vi "EX7-1_DC motor control.vi"() -> ()   [LabVIEW 2011]
uses:
  <vilib>/LabVIEW Interface for Arduino/LabVIEW Interface for Arduino.lvlib
panel:
  out "Ready?":bool
  in  "stop":bool
  in  "Selection":T1(radio)
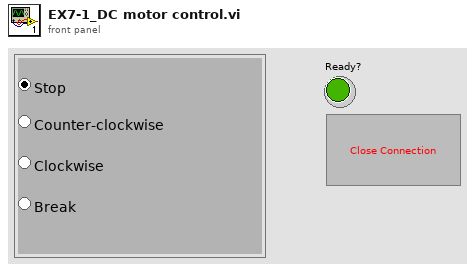
[diagram p1: front panel]
types:
  T1 = enum32{"Stop", "Clockwise", "Counter-clockwise", "Break"}
  T2 = typedef "LabVIEW Interface for Arduino.lvlib/Arduino Resource.ctl" = cluster{"VISA resource":refnum<visa-resource-name>, "Board Type":T3, "Connection Type":enum8{"USB / Serial"}, "Bytes Per Packet (15)":u8}
  T3 = typedef "LabVIEW Interface for Arduino.lvlib/Board Type.ctl" = enum16{"Uno", "Dimuelanove w/Atmega 328", "Mega 2560"}
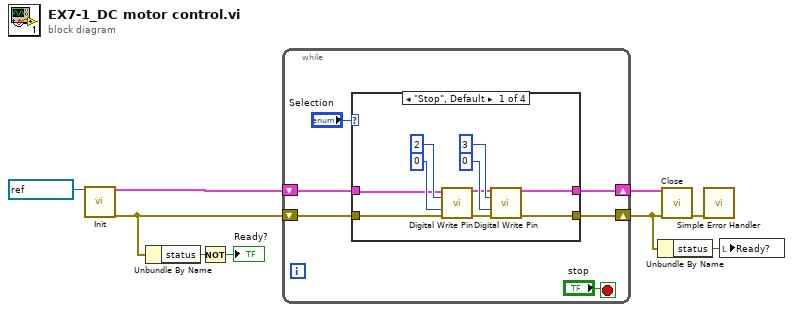
[diagram p0: block diagram]
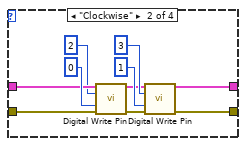
[diagram p2: hidden frame]
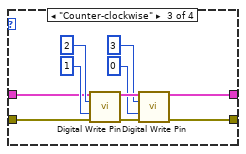
[diagram p3: hidden frame]
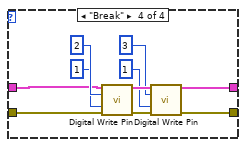
[diagram p4: hidden frame]
diagram:
  n1 = call <vilib>:"Init.vi"("VISA resource"=refnum<visa-resource-name> "COM9") -> ("Arduino Resource"=w8:T2, "error out"=w3:errorcluster)  [unwired: 17 in]
  n2 = Unbundle By Name(w3) -> ("status"=w4:bool)
  n3 = Not(x=w4) -> (.not. x?=→"Ready?":bool)
  n4 = while {
    shift-right: [w12] -> w7
    shift-left: w8 -> [w14]
    shift-right: [w11] -> w2
    shift-left: w3 -> [w13]
    stop <- "stop" stop-if-true
    n5 = case shown="\"Stop\", Default" "Selection" {
      tunnel: w14 -> [w20 w30 w39 w49]
      tunnel: w13 -> [w19 w29 w38 w48]
      tunnel: [w18 w28 w37 w47] -> w12
      tunnel: [w17 w27 w36 w46] -> w11
      frame "Stop", Default {
        n6 = call <vilib>:"Digital Write Pin.vi"("Arduino Resource"=w20, "Digital I/O Pin (0)"=u8 2, "Value (0)"=u8 0, "error in"=w19) -> ("Arduino Resource"=w16:T2, "error out"=w25:errorcluster)  [unwired: 10 in]
        n7 = call <vilib>:"Digital Write Pin.vi"("Arduino Resource"=w16, "Digital I/O Pin (0)"=u8 3, "Value (0)"=u8 0, "error in"=w25) -> ("Arduino Resource"=w18:T2, "error out"=w17:errorcluster)  [unwired: 10 in]
      }
      frame "Clockwise" {
        n8 = call <vilib>:"Digital Write Pin.vi"("Arduino Resource"=w30, "Digital I/O Pin (0)"=u8 2, "Value (0)"=u8 0, "error in"=w29) -> ("Arduino Resource"=w32:T2, "error out"=w31:errorcluster)  [unwired: 10 in]
        n9 = call <vilib>:"Digital Write Pin.vi"("Arduino Resource"=w32, "Digital I/O Pin (0)"=u8 3, "Value (0)"=u8 1, "error in"=w31) -> ("Arduino Resource"=w28:T2, "error out"=w27:errorcluster)  [unwired: 10 in]
      }
      frame "Counter-clockwise" {
        n10 = call <vilib>:"Digital Write Pin.vi"("Arduino Resource"=w39, "Digital I/O Pin (0)"=u8 2, "Value (0)"=u8 1, "error in"=w38) -> ("Arduino Resource"=w44:T2, "error out"=w45:errorcluster)  [unwired: 10 in]
        n11 = call <vilib>:"Digital Write Pin.vi"("Arduino Resource"=w44, "Digital I/O Pin (0)"=u8 3, "Value (0)"=u8 0, "error in"=w45) -> ("Arduino Resource"=w37:T2, "error out"=w36:errorcluster)  [unwired: 10 in]
      }
      frame "Break" {
        n12 = call <vilib>:"Digital Write Pin.vi"("Arduino Resource"=w49, "Digital I/O Pin (0)"=u8 2, "Value (0)"=u8 1, "error in"=w48) -> ("Arduino Resource"=w54:T2, "error out"=w55:errorcluster)  [unwired: 10 in]
        n13 = call <vilib>:"Digital Write Pin.vi"("Arduino Resource"=w54, "Digital I/O Pin (0)"=u8 3, "Value (0)"=u8 1, "error in"=w55) -> ("Arduino Resource"=w47:T2, "error out"=w46:errorcluster)  [unwired: 10 in]
      }
    }
  }
  n14 = Unbundle By Name(w2) -> ("status"=w1:bool)
  n15 = call <vilib>:"Close.vi"("Arduino Resource"=w7, "error in"=w2) -> ("error out"=w6:errorcluster)  [unwired: 13 in]
  n16 = call <vilib>:"Simple Error Handler.vi"("error in (no error)"=w6) -> ()  [unwired: 4 in, 5 out]
  n17 = local write "Ready?"(w1) -> ()
